vi "SP Update Formats on Measurement Changes.vi"(4 "error in (no error)":errorcluster, 6 "Parameter":T1, 7 "Format":refnum<vi>) -> (0 "error out":errorcluster)   [LabVIEW 2011]
uses:
  TypeDefs/MPSP Parameter.ctl
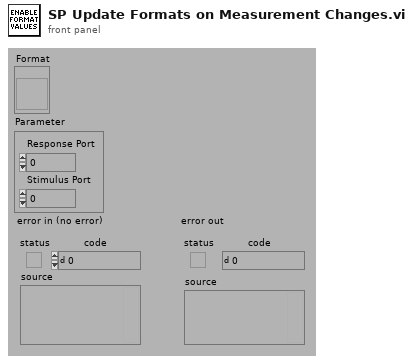
[diagram p1: front panel]
types:
  T1 = typedef "MPSP Parameter.ctl" = cluster{"Response Port":i8, "Stimulus Port":i8}
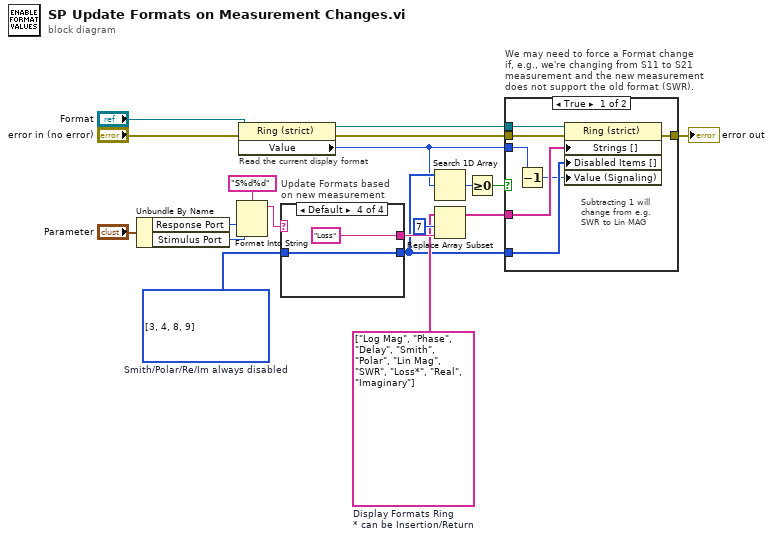
[diagram p0: block diagram]
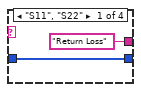
[diagram p2: hidden frame]
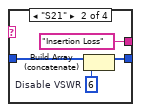
[diagram p3: hidden frame]
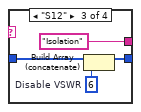
[diagram p4: hidden frame]
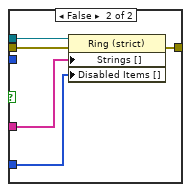
[diagram p5: hidden frame]
diagram:
  w12 = i32[] [3, 4, 8, 9]  # Smith/Polar/Re/Im always disabled
  w10 = string[] ["Log Mag", "Phase", "Delay", "Smith", "Polar", "Lin Mag", "SWR", "Loss*", "Real", "Imaginary"]  # Display Formats Ring * can be Insertion/Return
  # "Read the current display format"
  n1 = Unbundle By Name("Parameter") -> ("Response Port"=w4:i8, "Stimulus Port"=w3:i8)
  n2 = Format Into String(format string="S%d%d", w4, w3) -> (resulting string=w1:string)  [unwired: 2 in, 1 out]
  n3 = property on="Property Node" class="Ring (strict)"(reference="Format", error in="error in (no error)") -> (reference out=w19:refnum<vi>, error out=w17:errorcluster, "Value"=w6:i32)
  n4 = case "Update Formats based\non new measurement" shown="Default" w1 {
    tunnel: [w20 w24 w28 w30] -> w9
    tunnel: ["Return Loss" "Insertion Loss" "Isolation" "Loss"] -> w13
    tunnel: w12 -> [w20 w22 w26 w30]
    frame "S11", "S22" {
    }
    frame "S21" {
      w25 = 6  # Disable VSWR
      n5 = Build Array (concatenate)(w22, w25) -> (w24:i32[])
    }
    frame "S12" {
      w29 = 6  # Disable VSWR
      n6 = Build Array (concatenate)(w26, w29) -> (w28:i32[])
    }
    frame Default {
    }
  }
  n7 = Search 1D Array(1D array=w9, element=w6) -> (index of element=w8:i32)  [unwired: 1 in]
  n8 = Replace Array Subset(array=w10, new element=w13, index=7) -> (w11:string[])
  n9 = Greater Or Equal To 0?(x=w8) -> (x >= 0?=w7:bool)
  n10 = case "We may need to force a Format change\nif, e.g., we're changing from S11 to S21\nmeasurement and the new measurement\ndoes not support the old format (SWR)." shown="True" w7 {
    tunnel: w11 -> [w38 w43]
    tunnel: w19 -> [w37 w41]
    tunnel: [w36 w40] -> w18
    tunnel: w17 -> [w35 w42]
    tunnel: w9 -> [w34 w39]
    tunnel: w6 -> [w33 _]
    frame True {
      # "Subtracting 1 will\nchange from e.g.\nSWR to Lin MAG"
      n11 = Decrement(x=w33) -> (x-1=w32:i32)
      n12 = property on="Property Node" class="Ring (strict)"(reference=w37, error in=w35, "Strings []"=w38, "Disabled Items []"=w34, "Value (Signaling)"=w32) -> (error out=w36:errorcluster)  [unwired: 1 out]
    }
    frame False {
      n13 = property on="Property Node" class="Ring (strict)"(reference=w41, error in=w42, "Strings []"=w43, "Disabled Items []"=w39) -> (error out=w40:errorcluster)  [unwired: 1 out]
    }
  }
  "error out" <- w18
